vi "Elevator PID.vi"(10 "Button Pressed":dbl) -> ()   [LabVIEW 2014]
uses:
  Robot Global Data.vi
  <vilib>/addons/control/pid/pid.llb/PID (DBL).vi
  <vilib>/addons/control/pid/NI_PID_pid.lvlib
panel:
  out "Waveform Chart":dbl(graph)
  out "Motor Output":dbl
  out "Pot Value":dbl
  in  "PID gains":T1={"proportional gain (Kc)"=1.0, "integral time (Ti, min)"=0.01, "derivative time (Td, min)"=0.0} {"derivative time (Td, min)" format="%.3f"; "integral time (Ti, min)" format="%.3f"; "proportional gain (Kc)" format="%.3f"}
  # "5\n0.02\n0"
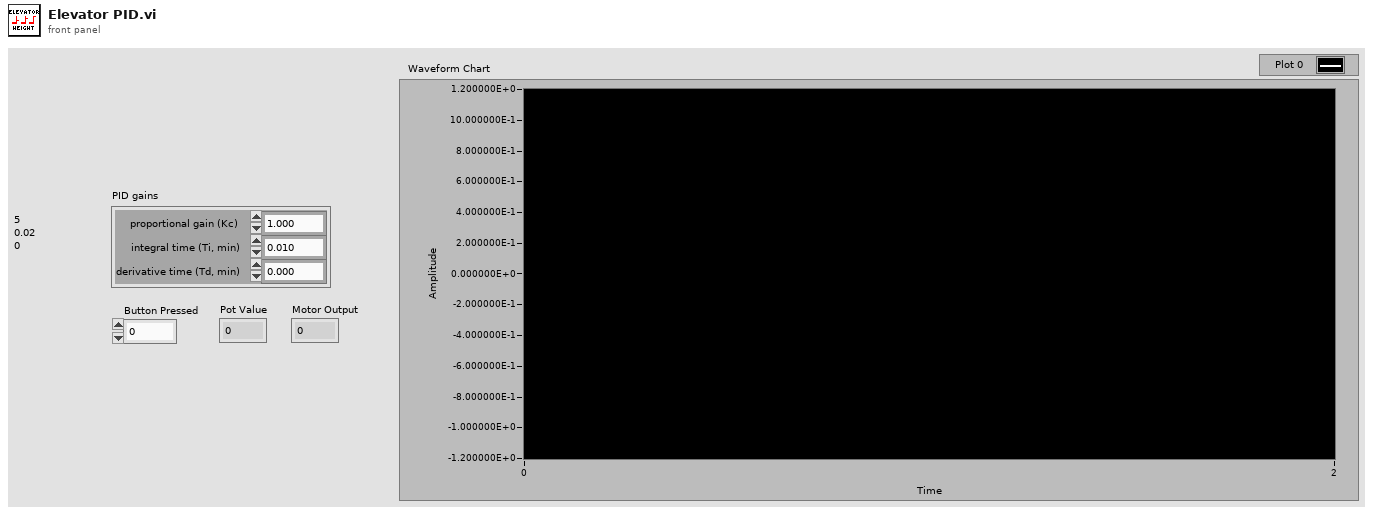
[diagram p1: front panel]
types:
  T1 = cluster{"proportional gain (Kc)":dbl, "integral time (Ti, min)":dbl, "derivative time (Td, min)":dbl}
  T2 = typedef "WPI_PotentiometerDevRef.ctl" = cluster{"DevStatus":errorcluster, "Controller":T3, "Analog Channel":T4, "Invert Output":bool}
  T3 = typedef "FPGA_TypedefAnalogModule.ctl" = enum16{"Controller 1"}
  T4 = typedef "FPGA_AIChannel.ctl" = enum8{"AI 0", "AI 1", "AI 2", "AI 3", "AI MXP 0", "AI MXP 1", "AI MXP 2", "AI MXP 3", "Invalid"}
  T5 = typedef "WPI_MotorControlDeviceRef.ctl" = cluster{"DeviceStatus":errorcluster, "Type":T6, "PWM":cluster{"Controller":T7, "PWM Channel":T8, "DeadBand":T9}, "CAN":cluster{"Device Number":u8, "Control Mode":T10, "Semaphore":T11, "Max Vout":dbl, "TalonSRX Control Mode":T12}, "Invert":bool, "TransformRef":T13, "InvTransformRef":T13}
  T6 = typedef "WPI_MotorControlType.ctl" = enum16{"PWM", "CAN", "CANTalonSRX"}
  T7 = typedef "FPGA_TypedefDigitalModule.ctl" = enum16{"Controller 1"}
  T8 = typedef "FPGA_DIOPWMChannel.ctl" = enum8{"PWM 0", "PWM 1", "PWM 2", "PWM 3", "PWM 4", "PWM 5", "PWM 6", "PWM 7", "PWM 8", "PWM 9", "PWM MXP 0", "PWM MXP 1", "PWM MXP 2", "PWM MXP 3", "PWM MXP 4", "PWM MXP 5", "PWM MXP 6", "PWM MXP 7", "PWM MXP 8", "PWM MXP 9", "Invalid"}
  T9 = typedef "WPI_PWMDeadband.ctl" = cluster{"Name":string, "maxPositivePwm":i32, "minPositivePwm":i32, "centerPwm":i32, "maxNegativePwm":i32, "minNegativePwm":i32, "angularRange":u16}
  T10 = typedef "WPI_CANJaguar_ControlMode.ctl" = enum8{"Percent VBus", "Current", "Speed", "Position", "Voltage"}
  T11 = typedef "Semaphore RefNum" = refnum<k1>
  T12 = typedef "WPI_CANTalonSRX_APIControlMode.ctl" = enum8{"Percent VBus", "Speed", "Position", "Slave", "Unchanged / Invalid"}
  T13 = typedef "WPI_PWMTransform_ConPane.ctl" = refnum<vi>
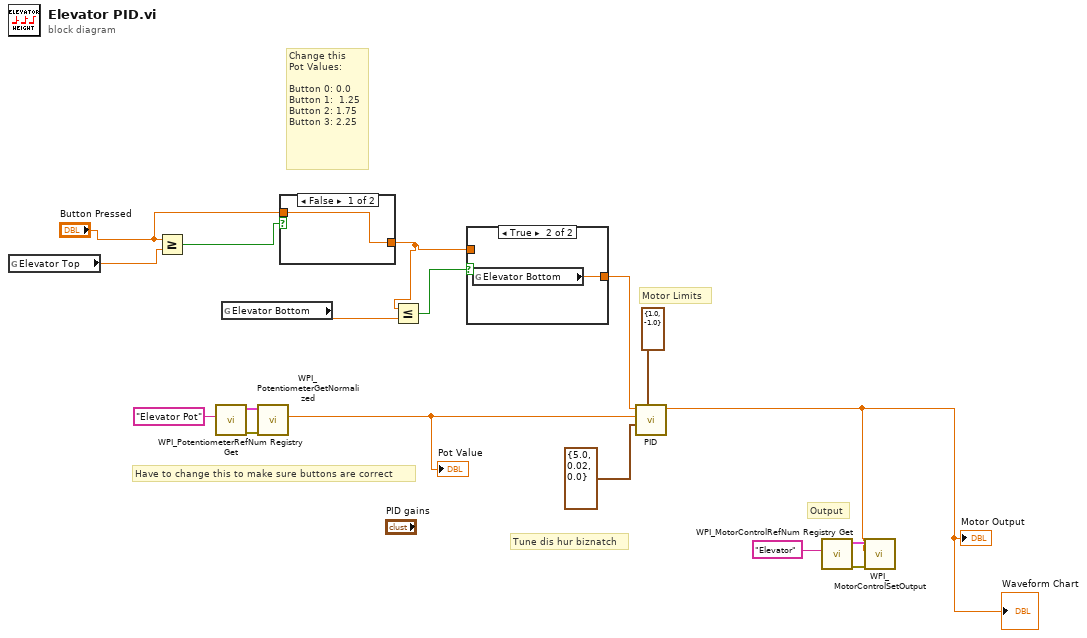
[diagram p0: block diagram]
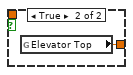
[diagram p3: hidden frame]
diagram:
  # "Output"
  # "Motor Limits"
  # "Tune dis hur biznatch"
  # "Change this \nPot Values:\n\nButton 0: 0.0\nButton 1:  1.25 \nButton 2: 1.75\nButton 3: 2.25"
  # "Have to change this to make sure buttons are correct"
  n1 = global read "Robot Global Data.vi" "Elevator Top"() -> (w7:dbl)
  n2 = Greater Or Equal?(x="Button Pressed", y=w7) -> (x >= y?=w6:bool)
  n3 = call <vilib>:"WPI_PotentiometerRefNum Registry Get.vi"("refnum name"="Elevator Pot") -> ("error out"=w17:errorcluster, "PotDevRef"=w16:T2)  [unwired: 9 in]
  n4 = global read "Robot Global Data.vi" "Elevator Bottom"() -> (w4:dbl)
  n5 = call <vilib>:"WPI_PotentiometerGetNormalized.vi"("error in"=w17, "PotDevRef"=w16) -> ("Normalized Value"=w10:dbl)  [unwired: 7 in, 2 out]
  "Pot Value" <- w10
  n6 = case shown="False" w6 {
    tunnel: [w18 w19] -> w2
    tunnel: "Button Pressed" -> [w18 _]
    frame False {
    }
    frame True {
      n7 = global read "Robot Global Data.vi" "Elevator Top"() -> (w19:dbl)
    }
  }
  n8 = Less Or Equal?(x=w2, y=w4) -> (x <= y?=w1:bool)
  n9 = case shown="True" w1 {
    tunnel: [w20 w21] -> w3
    tunnel: w2 -> [w20 _]
    frame False {
    }
    frame True {
      n10 = global read "Robot Global Data.vi" "Elevator Bottom"() -> (w21:dbl)
    }
  }
  n11 = call-poly <vilib>:"PID.vi"("output range"=cluster{"output high":dbl, "output low":dbl} {"output high"=1.0, "output low"=-1.0}, "PID gains"=T1 {"proportional gain (Kc)"=5.0, "integral time (Ti, min)"=0.02, "derivative time (Td, min)"=0.0}, "process variable"=w10, "setpoint"=w3) -> ("output"=w9:dbl)  [unwired: 6 in, 1 out]
  "Motor Output" <- w9
  "Waveform Chart" <- w9
  n12 = call <vilib>:"WPI_MotorControlRefNum Registry Get.vi"("refnum name"="Elevator") -> ("error out"=w15:errorcluster, "MotorControlDevRef"=w14:T5)  [unwired: 9 in]
  n13 = call <vilib>:"WPI_MotorControlSetOutput.vi"("error in (no error)"=w15, "Output"=w9, "MotorControlDevRef"=w14) -> ()  [unwired: 6 in, 3 out]
